vi "Check.vi"(9 "log line":string, 10 "current file":refnum<file>, 11 "size trigger in":refnum<class "RolloverTrigger.Size.lvclass">) -> (2 "rollover?":bool, 3 "size trigger out":refnum<class "RolloverTrigger.Size.lvclass">)   [LabVIEW 2018, in "GLog.lvlib" / "RolloverTrigger.Size.lvclass"]
doc: "Checks if the current file size exceeds the maximum file size."
uses:
  RolloverTrigger.Size.lvclass
  RolloverTrigger.Size.lvclass/RolloverTrigger.Size.ctl
panel:
  # "Connector Pane"
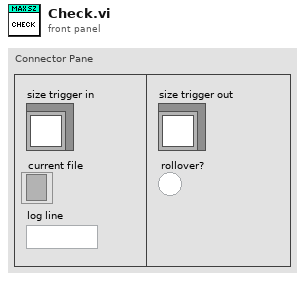
[diagram p1: front panel]
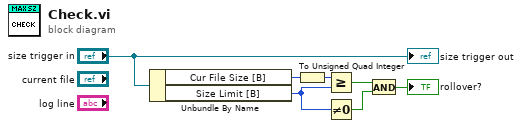
[diagram p0: block diagram]
diagram:
  n1 = Unbundle By Name("size trigger in") -> ("Cur File Size [B]"=w6:i64, "Size Limit [B]"=w3:u64)
  n2 = To Unsigned Quad Integer(1:w6) -> (0:w4:u64)
  n3 = Greater Or Equal?(x=w4, y=w3) -> (x >= y?=w7:bool)
  n4 = Not Equal To 0?(x=w3) -> (x != 0?=w1:bool)
  n5 = And(x=w7, y=w1) -> (x .and. y?=→"rollover?":bool)
  "size trigger out" <- "size trigger in"
